vi "Set configuration chain.vi"(8 "error in (no error)":errorcluster, 9 "class names":string[](array[string]), 10 "configuration":variant[](array[variant]), 11 "StageSPIM in":refnum<class "StageSPIM.lvclass">) -> (0 "error out":errorcluster, 3 "StageSPIM out":refnum<class "StageSPIM.lvclass">)   [LabVIEW 2012, in "StageSPIM.lvclass"]
uses:
  StageSPIM.lvclass
  <vilib>/Distrio/Murmex/Murmex/Murmex.lvclass
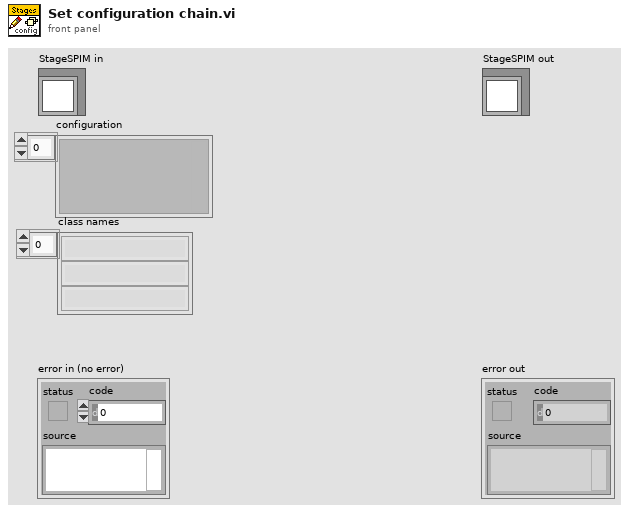
[diagram p1: front panel]
types:
  T1 = typedef "StageSPIM.lvclass/configuration_cluster.ctl" = cluster{"Port":T2, "Baudrate":T3, "Update frequency":dbl[unit], "S/N Master controller":string, "Interface":T4, "soft min limit":dbl[], "soft max limit":dbl[], "startup speedA":dbl[unit], "startup speedX":dbl[unit], "startup speedY":dbl[unit], "startup speedZ":dbl[unit], "startup speedFocus":dbl[unit], "autofocus ID":string}
  T2 = typedef "StageSPIM.lvclass/port_control.ctl" = i32
  T3 = typedef "StageSPIM.lvclass/baud_rate_control.ctl" = u16
  T4 = typedef "StageSPIM.lvclass/connection_type.ctl" = enum16{"RS232", "RS232 DaisyChain", "USB", "USB_DaisyChain"}
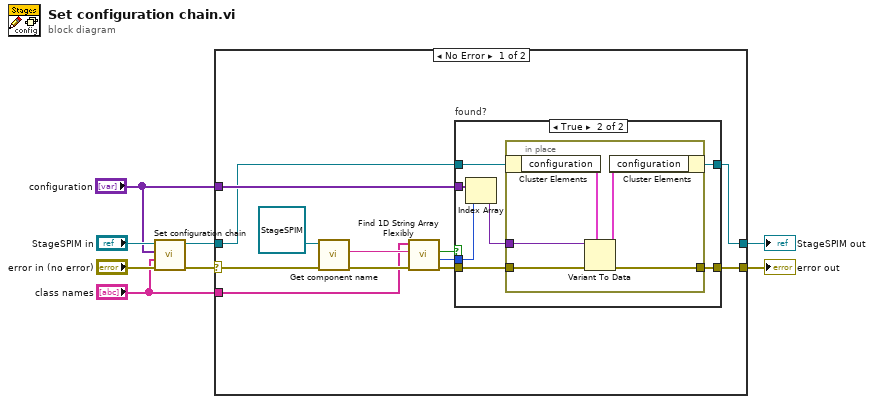
[diagram p0: block diagram]
diagram:
  n1 = call-parent "Set configuration chain.vi"("error in (no error)"="error in (no error)", "class names"="class names", "configuration"="configuration", "Murmex in"="StageSPIM in") -> ("error out"=w6:errorcluster, "Murmex out"=w3:refnum<class "StageSPIM.lvclass">)  [unwired: 6 in]
  n2 = case shown="No Error" w6 {
    selector: w6 -> [w14 w36]
    tunnel: [w15 w36] -> w5
    tunnel: [w9 w35] -> w4
    tunnel: w3 -> [w11 w35]
    tunnel: "class names" -> [w13 _]
    tunnel: "configuration" -> [w12 _]
    frame No Error {
      n3 = call <vilib>:"Get component name.vi"("error in (no error)"=w14, "Murmex in"=refnum<class "StageSPIM.lvclass"> refnum ("StageSPIM in")) -> ("error out"=w20:errorcluster, "component name"=w18:string)  [unwired: 7 in, 1 out]
      n4 = call <vilib>:"Find 1D String Array Flexibly.vi"("error in (no error)"=w20, "element"=w18, "array"=w13) -> ("error out"=w19:errorcluster, "index of element"=w17:i32, "found?"=w16:bool)  [unwired: 6 in]
      n5 = case "found?" shown="True" w16 {
        tunnel: w12 -> [_ w29]
        tunnel: w11 -> [w22 w27]
        tunnel: [w22 w26] -> w9
        tunnel: [w21 w25] -> w15
        tunnel: w19 -> [w21 w24]
        tunnel: w17 -> [_ w23]
        frame False {
        }
        frame True {
          n6 = Index Array(array=w29, index=w23) -> (element=w28:variant)
          n7 = in-place {
            in-place-border: w28 -> [w34]
            in-place-border: w24 -> [w32]
            in-place-border: [w30] -> w25
            n8 = in-place-cluster #1(w27) -> ("configuration"=w33:T1)
            n9 = Variant To Data(error in=w32, type=w33, Variant=w34) -> (data=w31:T1, error out=w30:errorcluster)
            n10 = in-place-cluster #1("configuration"=w31) -> (w26:refnum<class "StageSPIM.lvclass">)
          }
        }
      }
    }
    frame Error {
    }
  }
  "error out" <- w5
  "StageSPIM out" <- w4
